vi "动态刷新波形图表.vi"() -> ()   [LabVIEW 2014]
panel:
  out "波形图表":T1(graph)
  in  "布尔":bool
  in  "停止":bool
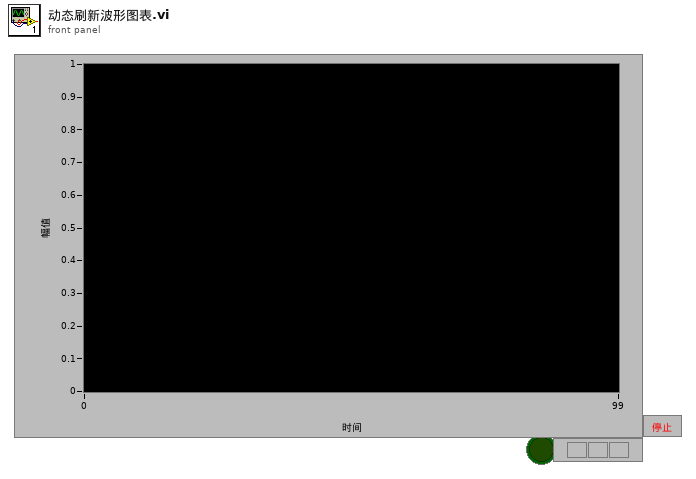
[diagram p1: front panel]
types:
  T1 = cluster{"number: 0 to 1":dbl, "number: 0 to 1":dbl}[]
  T2 = cluster{"number: 0 to 1":dbl, "number: 0 to 1":dbl}
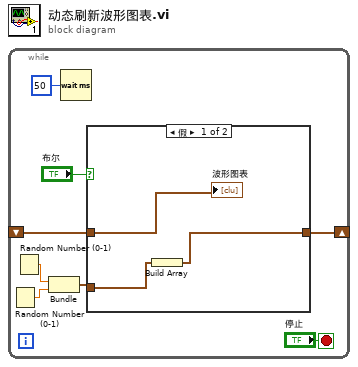
[diagram p0: block diagram]
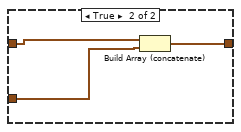
[diagram p2: hidden frame]
diagram:
  n1 = while {
    shift-right: [w2] -> _
    shift-left: _ -> [w1]
    stop <- "停止" stop-if-true
    n2 = Random Number (0-1)() -> (number: 0 to 1=w5:dbl)
    n3 = Random Number (0-1)() -> (number: 0 to 1=w4:dbl)
    n4 = Bundle("number: 0 to 1"=w4, "number: 0 to 1"=w5) -> (w3:T2)  [unwired: 1 in]
    n5 = Wait (ms)(milliseconds to wait=u32 50 ("等待时间（毫秒）")) -> ()  [unwired: 1 out]
    n6 = case shown="假" "布尔" {
      tunnel: w3 -> [w11 w13]
      tunnel: [w10 w14] -> w2
      tunnel: w1 -> [w9 w12]
      frame False {
        n7 = Build Array(w11) -> (w10:T1)
        "波形图表" <- w9
      }
      frame True {
        n8 = Build Array (concatenate)(w12, w13) -> (w14:T1)
      }
    }
  }
